vi "Query with Scalar 64bit Integer Result.vi"(8 "error in (no error)":errorcluster, 10 "Query string":string, 11 "sqlite3 in":refnum<class "sqlite3.lvclass">) -> (0 "error out":errorcluster, 2 "Result":i64, 3 "sqlite3 out":refnum<class "sqlite3.lvclass">)   [LabVIEW 2020, in "sqlite3.lvlib" / "sqlite3.lvclass"]
uses:
  sqlite3.lvclass
  sqlite3.lvclass/sqlite3.ctl
  a697d987-ad6e-4e1d-929a-601234a1e2d4.vi
  sqlite/VIs/open v2.vi
  sqlite/VIs/close v2.vi
  sqlite/VIs/prepare v2.vi
  sqlite/VIs/step.vi
  sqlite/VIs/column count.vi
  db layer/compound/Resolve Result Type.vi
  a697d987-ad6e-4e1d-929a-601234a1e2d4.vi/0244caef-bc9a-4150-a8ac-bf3d364b181c.vi
  a697d987-ad6e-4e1d-929a-601234a1e2d4.vi/5568208c-18c9-421a-afbc-e39208249946.vi
  sqlite/VIs/finalize.vi
  sqlite/subvi/Error Converter (ErrCode or Status).vi
  sqlite/VIs/column type.vi
  sqlite/VIs/column int64.vi
  a697d987-ad6e-4e1d-929a-601234a1e2d4.vi/0244caef-bc9a-4150-a8ac-bf3d364b181c.vi/c3a74749-1ef8-497f-bac9-7930eb10c389.vi
  a697d987-ad6e-4e1d-929a-601234a1e2d4.vi/5568208c-18c9-421a-afbc-e39208249946.vi/75192634-ebc5-405e-9af9-59334ea50174.vi
  sqlite/VIs/errstr.vi
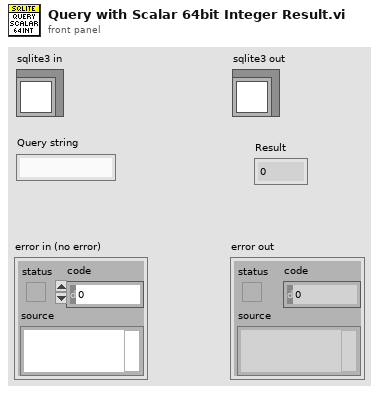
[diagram p1: front panel]
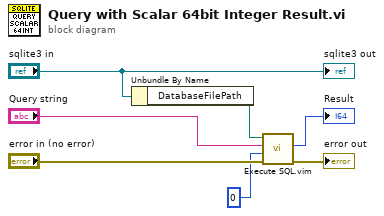
[diagram p0: block diagram]
diagram:
  n1 = Unbundle By Name("sqlite3 in") -> ("DatabaseFilePath"=w7:path)
  n2 = call "Execute SQL.vim"("error in (no error)"="error in (no error)", "desired return type(none)"=i64 0, "sql (string)"="Query string", "database in"=w7) -> ("error out"=→"error out":errorcluster, "Query Result"=→"Result":i64)  [unwired: 6 in]
  "sqlite3 out" <- "sqlite3 in"
